vi "Finalize.vi"(8 "error in":errorcluster, 11 "Monitor Execution Unit in":refnum<class "Monitor Execution Unit.lvclass">) -> (0 "error out":errorcluster, 3 "Monitor Execution Unit out":refnum<class "Monitor Execution Unit.lvclass">)   [LabVIEW 2020, in "AIM ARINC 664 Engine.lvlib" / "Implementation.lvlib" / "Monitor Execution Unit.lvclass"]
uses:
  Monitor Execution Unit.lvclass
  Monitor Execution Unit.lvclass/Monitor Execution Unit.ctl
  <instrlib>/AIM GmbH/_AIM 664/bsp/Fdx Stop (Rx).vi
  <instrlib>/AIM GmbH/_AIM 664/AIM664LV.lvlib
  Logging/Frame Logging/Frame Logging.lvlib
  <vilib>/Utility/SystemLogging/NI_SystemLogging.lvlib
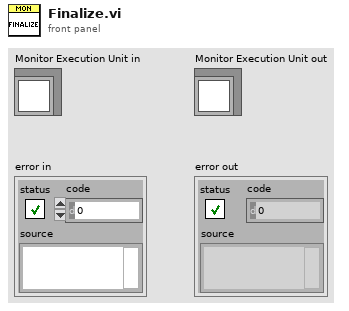
[diagram p1: front panel]
types:
  T1 = typedef "Frame Logging.lvlib/Log_Producer.ctl" = cluster{"Configured":bool, "message queue in":refnum<queue>, "StopNotification":refnum<notifier>}
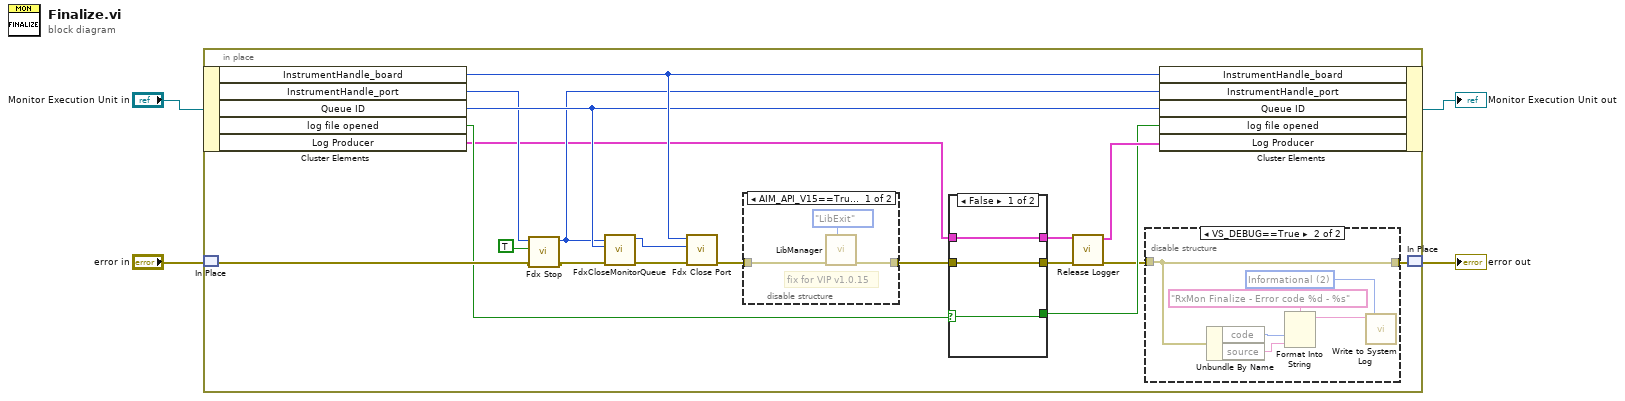
[diagram p0: block diagram]
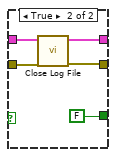
[diagram p4: hidden frame]
diagram:
  n1 = in-place {
    n2 = in-place-cluster #1("Monitor Execution Unit in") -> ("InstrumentHandle_board"=w23:u32, "InstrumentHandle_port"=w19:u32, "Queue ID"=w20:u32, "log file opened"=w14:bool, "Log Producer"=w13:T1)
    n3 = in-place-match #2("error in") -> (w17:errorcluster)
    n4 = call-poly <instrlib>:"Fdx Stop.vi"("error in"=w17, "Force Stop?"=TRUE, "InstrumentHandle_port in"=w19) -> ("error out"=w16:errorcluster, "InstrumentHandle_port out"=w15:u32)  [unwired: 7 in]
    n5 = call <instrlib>:"FdxCloseMonitorQueue.vi"("error in"=w16, "QueueId"=w20, "InstrumentHandle_port in"=w15) -> ("error out"=w22:errorcluster, "InstrumentHandle_port out"=w21:u32)  [unwired: 7 in]
    n6 = call <instrlib>:"Fdx Close Port.vi"("error in"=w22, "InstrumentHandle_port in"=w21, "InstrumentHandle_board in"=w23) -> ("error out"=w8:errorcluster)  [unwired: 7 in, 1 out]
    n7 = disable-structure shown="AIM_API_V15==True" {
      disable-tunnel: w8 -> [w33 w34]
      disable-tunnel: [w32 w34] -> w7
      frame condition #0 {
        # "fix for VIP v1.0.15"
        n8 = call <instrlib>:"LibManager.vi"("action"=enum16{"LibInit", "LibExit"}."LibExit", "error in (no error)"=w33) -> ("error out"=w32:errorcluster)  [unwired: 7 in, 2 out]
      }
      frame condition #1 (active) {
      }
    }
    n9 = case shown="False" w14 {
      selector: w14 -> [w35 _]
      tunnel: [w37 w41] -> w10
      tunnel: w7 -> [w37 w42]
      tunnel: w13 -> [w36 w40]
      tunnel: [w36 w39] -> w11
      tunnel: [w35 FALSE] -> w9
      frame False {
      }
      frame True {
        n10 = call "Close Log File.vi"("error in"=w42, "Log Producer in"=w40) -> ("error out"=w41:errorcluster, "Log Producer out"=w39:T1)  [unwired: 8 in]
      }
    }
    n11 = call "Release Logger.vi"("error in (no error)"=w10, "Log Producer in"=w11) -> ("error out"=w6:errorcluster, "Log Producer out"=w12:T1)  [unwired: 8 in]
    n12 = disable-structure shown="VS_DEBUG==True" {
      disable-tunnel: w6 -> [w24 w25]
      disable-tunnel: [w24 w25] -> w5
      frame condition #0 (active) {
      }
      frame condition #1 {
        w28 = 2 items=["Error", "Warning", "Informational"] ("severity")
        n13 = Unbundle By Name(w25) -> ("code"=w27:i32, "source"=w26:string)
        n14 = Format Into String(format string="RxMon Finalize - Error code %d - %s", w27, w26) -> (resulting string=w29:string)  [unwired: 2 in, 1 out]
        n15 = call <vilib>:"Write to System Log.vi"("severity"=w28, "message"=w29) -> ()  [unwired: 9 in, 1 out]
      }
    }
    n16 = in-place-cluster #1("InstrumentHandle_board"=w23, "InstrumentHandle_port"=w15, "Queue ID"=w20, "log file opened"=w9, "Log Producer"=w12) -> (→"Monitor Execution Unit out":refnum<class "Monitor Execution Unit.lvclass">)
    n17 = in-place-match #2(w5) -> (→"error out":errorcluster)
  }
